vi "Make Project Copy.vi"(8 "error in (no error)":errorcluster, 11 "UI Data":T1) -> (0 "error out":errorcluster, 1 "Cancelled":bool, 2 "Name out":string, 3 "Project Root Path":path)   [LabVIEW 2013, in "Project Wizard.lvlib"]
uses:
  Project Wizard.lvlib
  controls/UI Data.ctl
  controls/Template.ctl
  support/Alert Dialogs/Dlg Symbol.ctl
  support/Alert Dialogs/Dlg Button.ctl
  support/Alert Dialogs/Alert Dialogs.lvlib
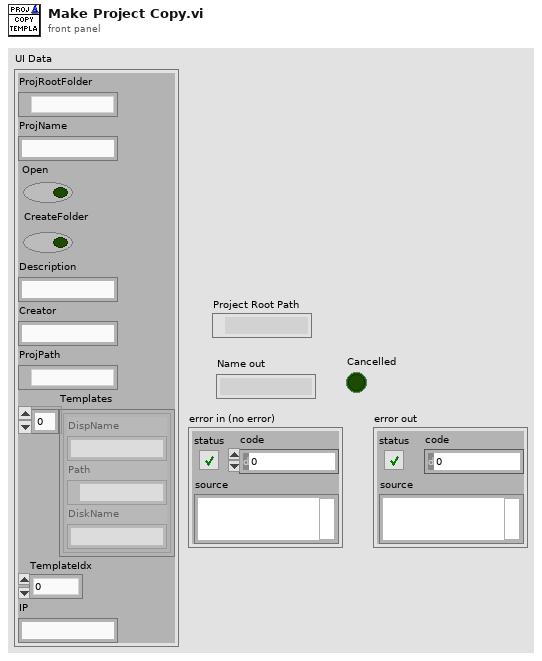
[diagram p1: front panel]
types:
  T1 = typedef "Project Wizard.lvlib/UI Data.ctl" = cluster{"ProjRootFolder":path, "ProjName":string, "Open":bool, "CreateFolder":bool, "Description":string, "Creator":string, "ProjPath":path, "Templates":T2[], "TemplateIdx":u16, "IP":string}
  T2 = typedef "Project Wizard.lvlib/Template.ctl" = cluster{"DispName":string, "Path":path, "DiskName":string}
  T3 = typedef "Project Wizard.lvlib/Alert Dialogs.lvlib/Dlg Symbol.ctl" = enum16{"Information", "Help", "Warning", "Error"}
  T4 = cluster{"Focus":bool, "Control":bool, "Shift":bool, "Key":string}[]
  T5 = typedef "Project Wizard.lvlib/Alert Dialogs.lvlib/Dlg Button.ctl" = enum16{"Left Button", "Center Button", "Right Button", "Window Close"}
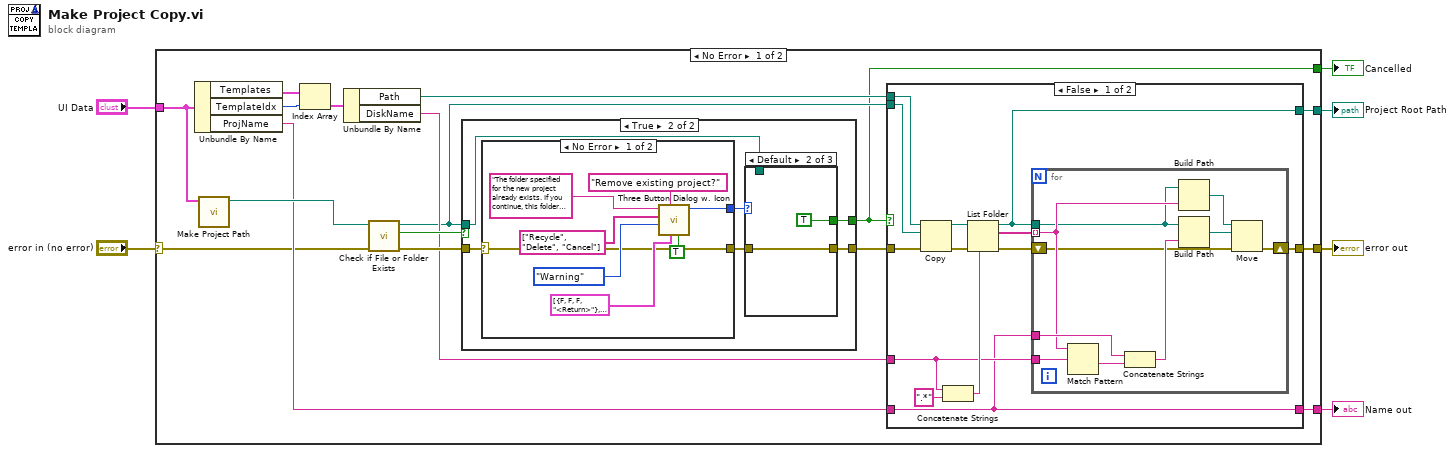
[diagram p0: block diagram]
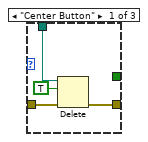
[diagram p4: hidden frame]
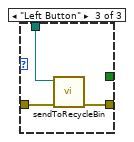
[diagram p5: hidden frame]
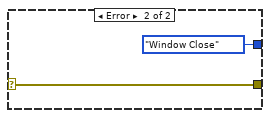
[diagram p6: hidden frame]
diagram:
  n1 = case shown="No Error" "error in (no error)" {
    selector: "error in (no error)" -> [w10 w74]
    tunnel: [w23 w74] -> w6
    tunnel: [w22 _] -> w5
    tunnel: "UI Data" -> [w14 _]
    tunnel: [w8 _] -> w2
    tunnel: [w7 _] -> w1
    frame No Error {
      n2 = Unbundle By Name(w14) -> ("Templates"=w18:T2[], "TemplateIdx"=w17:u16, "ProjName"=w11:string)
      n3 = call "Make Project Path.vi"("Data Cluster"=w14) -> ("project folder"=w13:path)  [unwired: 9 in, 1 out]
      n4 = Index Array(array=w18, index=w17) -> (element=w16:T2)
      n5 = Unbundle By Name(w16) -> ("Path"=w15:path, "DiskName"=w12:string)
      n6 = call <vilib>:"Check if File or Folder Exists.vi"("error in (no error)"=w10, "path"=w13) -> ("error out"=w20:errorcluster, "file or folder exists?"=w21:bool, "dup path"=w9:path)  [unwired: 7 in]
      n7 = case shown="True" w21 {
        tunnel: w20 -> [w48 w53]
        tunnel: [w48 w54] -> w19
        tunnel: w9 -> [_ w50]
        tunnel: [_ w49] -> w8
        frame False {
        }
        frame True {
          n8 = case shown="No Error" w53 {
            selector: w53 -> [w65 w73]
            tunnel: [w65 w73] -> w52
            tunnel: [w64 Dlg_Button."Window Close" ("Which Button?")] -> w51
            frame No Error {
              n9 = call "Three Button Dialog w. Icon.vi"("Allow User to Close Dialog (T)"=TRUE, "Toggle Key Shortcut (<Return>, , <Esc>"=T4 [{"Focus"=FALSE, "Control"=FALSE, "Shift"=FALSE, "Key"="<Return>"}, {"Focus"=FALSE, "Control"=FALSE, "Shift"=FALSE, "Key"=""}, {"Focus"=FALSE, "Control"=FALSE, "Shift"=FALSE, "Key"="<Escape>"}], "Window Title (\"\")"="Remove existing project?" ("Window Title (\"\")"), "Symbol"=Dlg_Symbol."Warning", "Button Strings"=string[] ["Recycle", "Delete", "Cancel"], "Message"="The folder specified for the new project already exists. If you continue, this folder must be removed. Recycle or delete it?") -> ("Which Button?"=w64:T5)  [unwired: 5 in]
            }
            frame Error {
            }
          }
          n10 = case shown="Default" w51 {
            tunnel: [w57 w60 w63] -> w54
            tunnel: w52 -> [w58 w60 w62]
            tunnel: w50 -> [w56 _ w61]
            tunnel: [_ TRUE _] -> w49
            frame "Center Button" {
              n11 = Delete(path (use dialog)=w56, entire hierarchy (F)=TRUE, error in=w58) -> (error out=w57:errorcluster)  [unwired: 2 in, 2 out]
            }
            frame Default {
            }
            frame "Left Button" {
              n12 = call "sendToRecycleBin.vi"("error in"=w62, "Directory to Recycle"=w61) -> ("error out"=w63:errorcluster)  [unwired: 9 in]
            }
          }
        }
      }
      n13 = case shown="False" w8 {
        tunnel: [w36 w47] -> w23
        tunnel: [w35 _] -> w22
        tunnel: w19 -> [w30 w47]
        tunnel: w15 -> [w27 _]
        tunnel: w12 -> [w26 _]
        tunnel: w11 -> [w24 _]
        tunnel: w9 -> [w25 _]
        tunnel: [w24 _] -> w7
        frame False {
          n14 = Copy(8:w30, 10:w25, 11:w27) -> (0:w33:errorcluster, 3:w34:path)  [unwired: 2 in, 1 out]
          n15 = Concatenate Strings(w26, ".*" ("string")) -> (w28:string)
          n16 = List Folder(path=w34, pattern=w28, error in=w33) -> (path out=w35:path, filenames=w32:string[], error out=w31:errorcluster)  [unwired: 1 in, 1 out]
          n17 = for {
            tunnel: w32 -> [w43] mode=indexing
            shift-right: [w39] -> w36
            shift-left: w31 -> [w40]
            tunnel: w24 -> [w46]
            tunnel: w26 -> [w37]
            tunnel: w35 -> [w38]
            n18 = Match Pattern(string=w43, regular expression=w37) -> (after substring=w45:string)  [unwired: 1 in, 3 out]
            n19 = Concatenate Strings(w46, w45) -> (w44:string)
            n20 = Build Path(base path=w38, name or relative path=w43) -> (appended path=w42:path)
            n21 = Build Path(base path=w38, name or relative path=w44) -> (appended path=w41:path)
            n22 = Move(source path=w42, error in=w40, 10:w41) -> (error out=w39:errorcluster)  [unwired: 2 in, 2 out]
          }
        }
        frame True {
        }
      }
    }
    frame Error {
    }
  }
  "error out" <- w6
  "Project Root Path" <- w5
  "Cancelled" <- w2
  "Name out" <- w1
